vi "p2.vi"() -> ()   [LabVIEW 2023, in "d15.lvlib"]
uses:
  d15.lvlib
  <vilib>/Utility/miscctls.llb/LVMapReplaceAction.ctl
  AOC/AOC.lvlib
panel:
  in  "Example":string="rn=1,cm-,qp=3,cm=2,qp-,pc=4,ot=9,ab=5,pc-,pc=6,ot=7"
  in  "Example":bool
  out "Answer":u64=4737443
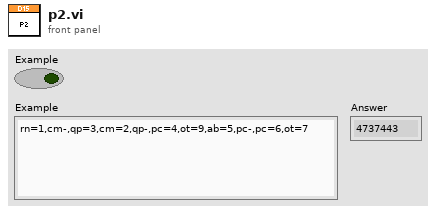
[diagram p1: front panel]
types:
  T1 = map{string, cluster{"Focal Length":u8, "Position":u16}}
  T2 = map{string, cluster{"Focal Length":u8, "Position":u16}}[]
  T3 = typedef "LVMapReplaceAction.ctl" = enum32{"Modify Entry only if found", "Add or Modify Entry", "Delete Entry"}
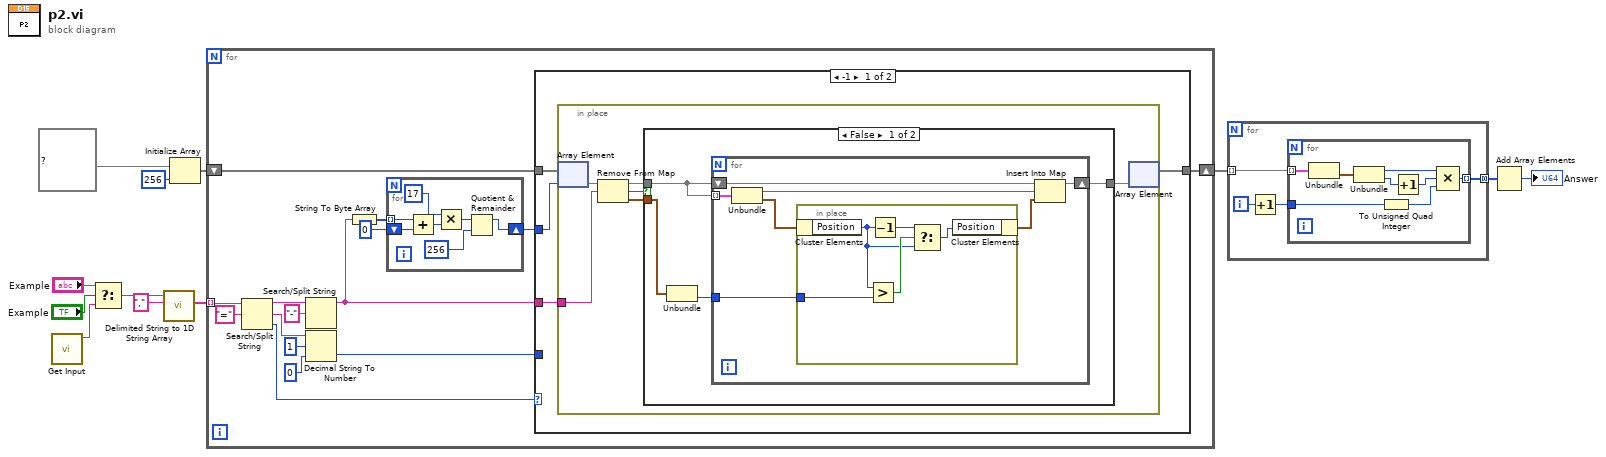
[diagram p0: block diagram]
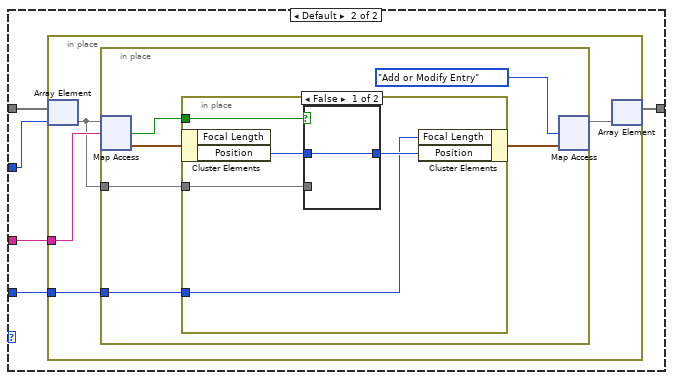
[diagram p3: hidden frame]
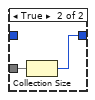
[diagram p4: hidden frame]
diagram:
  n1 = call "Get Input.vi"() -> ("Input"=w12:string)  [unwired: 11 in]
  n2 = Select(t="Example", s="Example", f=w12) -> (s? t:f=w2:string)
  n3 = call <vilib>:"Delimited String to 1D String Array.vi"("delimiter"=",", "delimited string"=w2) -> ("string array"=w9:string[])  [unwired: 9 in]
  n4 = Initialize Array(T1 {} ("Map"), 256 ("dimension size")) -> (w6:T2)
  n5 = for {
    tunnel: w9 -> [w24] mode=indexing
    shift-right: [w17] -> w4
    shift-left: w6 -> [w20]
    n6 = Search/Split String(string=w24, search string/char (-)="=") -> (substring before match=w23:string, match + rest of string=w16:string, offset of match=w21:i32)  [unwired: 1 in]
    n7 = Search/Split String(string=w23, search string/char (-)="-") -> (substring before match=w18:string)  [unwired: 1 in, 2 out]
    n8 = Decimal String To Number(string=w16, offset=1, default (0L)=u8 0 ("default (0 I32)")) -> (number=w15:u8)  [unwired: 1 out]
    n9 = String To Byte Array(string=w18) -> (unsigned byte array=w26:u8[])
    n10 = for {
      shift-right: [w78] -> w19
      shift-left: u64 0 -> [w84]
      tunnel: w26 -> [w83] mode=indexing
      n11 = Add(x=w83, y=w84) -> (x+y=w82:u64)
      n12 = Multiply(x=u64 17, y=w82) -> (x*y=w80:u64)
      n13 = Quotient & Remainder(x=w80, y=u64 256) -> (x-y*floor(x/y)=w78:u64)  [unwired: 1 out]
    }
    n14 = case shown="-1" w21 {
      tunnel: w20 -> [w31 w58]
      tunnel: w19 -> [w30 w57]
      tunnel: w18 -> [w28 w59]
      tunnel: [w29 w56] -> w17
      tunnel: w15 -> [_ w55]
      frame -1 {
        n15 = in-place {
          in-place-border: w28 -> [w36]
          n16 = in-place-array #1(w31, w30) -> (w37:T1)
          n17 = Remove From Map(10:w36, 11:w37) -> (1:w35:cluster{"Focal Length":u8, "Position":u16}, 2:w32:bool, 3:w34:T1)
          n18 = case shown="False" w32 {
            tunnel: w35 -> [w41 _]
            tunnel: w34 -> [w39 w54]
            tunnel: [w38 w54] -> w33
            frame False {
              n19 = Unbundle(w41) -> ("Position"=w40:u16)  [unwired: 1 out]
              n20 = for {
                tunnel: w39 -> [w48] mode=indexing
                tunnel: w40 -> [w42]
                shift-right: [w46] -> w38
                shift-left: w39 -> [w47]
                n21 = Unbundle(w48) -> ("substring before match"=w45:string, w44:cluster{"Focal Length":u8, "Position":u16})
                n22 = in-place {
                  in-place-border: w42 -> [w49]
                  n23 = in-place-cluster #2(w44) -> ("Position"=w51:u16)
                  n24 = Greater?(x=w51, y=w49) -> (0:w52:bool)
                  n25 = Decrement(x=w51) -> (x-1=w53:u16)
                  n26 = Select(t=w53, s=w52, f=w51) -> (s? t:f=w50:u16)
                  n27 = in-place-cluster #2("Position"=w50) -> (w43:cluster{"Focal Length":u8, "Position":u16})
                }
                n28 = Insert Into Map(map in=w47, key=w45, value=w43) -> (map out=w46:T1)  [unwired: 2 out]
              }
            }
            frame True {
            }
          }
          n29 = in-place-array #1(w33) -> (w29:T2)  [unwired: 1 out]
        }
      }
      frame Default {
        n30 = in-place {
          in-place-border: w59 -> [w62]
          in-place-border: w55 -> [w63]
          n31 = in-place-array #3(w58, w57) -> (w60:T1)
          n32 = in-place {
            in-place-border: w63 -> [w69]
            in-place-border: w60 -> [w66]
            n33 = in-place-map #4(w60, w62) -> (w65:cluster{"Focal Length":u8, "Position":u16}, w68:bool)  [unwired: 1 in]
            n34 = in-place {
              in-place-border: w69 -> [w70]
              in-place-border: w68 -> [w74]
              in-place-border: w66 -> [w73]
              n35 = in-place-cluster #5(w65) -> ("Position"=w72:u16)  [unwired: 1 out]
              n36 = case shown="False" w74 {
                tunnel: w73 -> [_ w77]
                tunnel: w72 -> [w75 _]
                tunnel: [w75 w76] -> w71
                frame False {
                }
                frame True {
                  n37 = Collection Size(1:w77) -> (0:w76:i32)
                }
              }
              n38 = in-place-cluster #5("Focal Length"=w70, "Position"=w71) -> (w64:cluster{"Focal Length":u8, "Position":u16})
            }
            n39 = in-place-map #4(w64, LVMapReplaceAction."Add or Modify Entry" ("action")) -> (w61:T1)  [unwired: 2 out]
          }
          n40 = in-place-array #3(w61) -> (w56:T2)  [unwired: 1 out]
        }
      }
    }
  }
  n41 = for {
    tunnel: w4 -> [w88] mode=indexing
    tunnel: [w85] -> w3 mode=concatenating
    i -> [w87]
    n42 = Increment(x=w87) -> (x+1=w86:i32)
    n43 = for {
      tunnel: w88 -> [w96] mode=indexing
      tunnel: w86 -> [w93]
      tunnel: [w92] -> w85 mode=indexing
      n44 = Unbundle(w96) -> (w95:cluster{"Focal Length":u8, "Position":u16})  [unwired: 1 out]
      n45 = Unbundle(w95) -> ("Focal Length"=w91:u8, "Position"=w94:u16)
      n46 = To Unsigned Quad Integer(1:w93) -> (0:w89:u64)
      n47 = Increment(x=w94) -> (x+1=w90:u16)
      n48 = Compound Arithmetic op=MULTIPLY(w91, w90, w89) -> (w92:u64)
    }
  }
  n49 = Add Array Elements(numeric array=w3) -> (sum=→"Answer":u64)
